vi "verificarDatosProducto.vi"(8 "error in":errorcluster, 11 "dataToWrite":T2) -> (0 "error out":errorcluster, 3 "dataToWriteModify":T1)   [LabVIEW 2014]
uses:
  <vilib>/addons/database/Auxilliary.llb/DB Tools Format Datetime String (Time Stamp).vi
  <vilib>/addons/database/NI_Database_API.lvlib
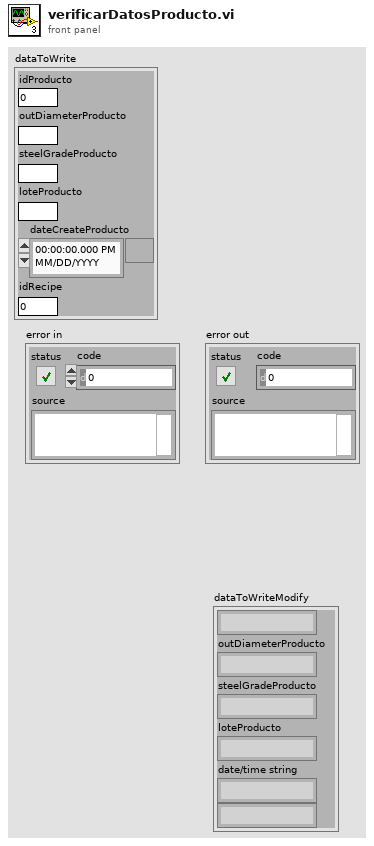
[diagram p1: front panel]
types:
  T1 = cluster{string, "outDiameterProducto":string, "steelGradeProducto":string, "loteProducto":string, "date/time string":string, string}
  T2 = cluster{"idProducto":dbl, "outDiameterProducto":string, "steelGradeProducto":string, "loteProducto":string, "dateCreateProducto":timestamp, "idRecipe":dbl}
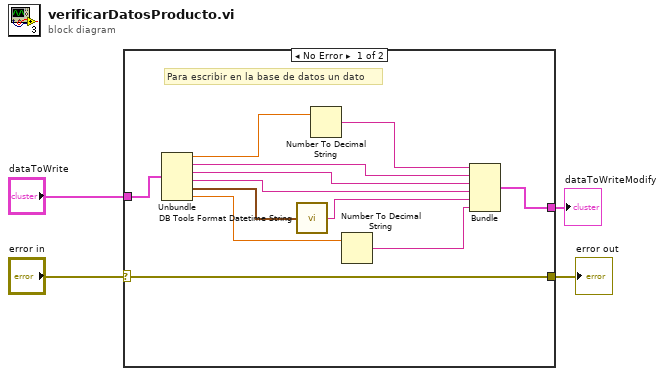
[diagram p0: block diagram]
diagram:
  n1 = case shown="No Error" "error in" {
    selector: "error in" -> [w11 w17]
    tunnel: "dataToWrite" -> [w16 _]
    tunnel: [w15 _] -> w1
    tunnel: [w11 w17] -> w3
    frame No Error {
      # "Para escribir en la base de datos un dato"
      n2 = Unbundle(w16) -> ("idProducto"=w13:dbl, "outDiameterProducto"=w12:string, "steelGradeProducto"=w9:string, "loteProducto"=w8:string, "dateCreateProducto"=w10:timestamp, "idRecipe"=w6:dbl)
      n3 = call-poly <vilib>:"DB Tools Format Datetime String.vi"("time stamp"=w10) -> ("date/time string"=w7:string)
      n4 = Number To Decimal String(number=w13) -> (decimal integer string=w14:string)  [unwired: 1 in]
      n5 = Number To Decimal String(number=w6) -> (decimal integer string=w5:string)  [unwired: 1 in]
      n6 = Bundle(w14, "outDiameterProducto"=w12, "steelGradeProducto"=w9, "loteProducto"=w8, "date/time string"=w7, w5) -> (w15:T1)  [unwired: 1 in]
    }
    frame Error {
    }
  }
  "error out" <- w3
  "dataToWriteModify" <- w1
